vi "Write B.vi"(8 "error in (no error)":errorcluster, 10 "B":dbl, 11 "NumericOperation in":refnum<class "NumericOperation.lvclass">) -> (0 "error out":errorcluster, 3 "NumericOperation out":refnum<class "NumericOperation.lvclass">)   [LabVIEW 2021, in "Calculator.lvlib" / "NumericOperation.lvclass"]
uses:
  NumericOperation.lvclass
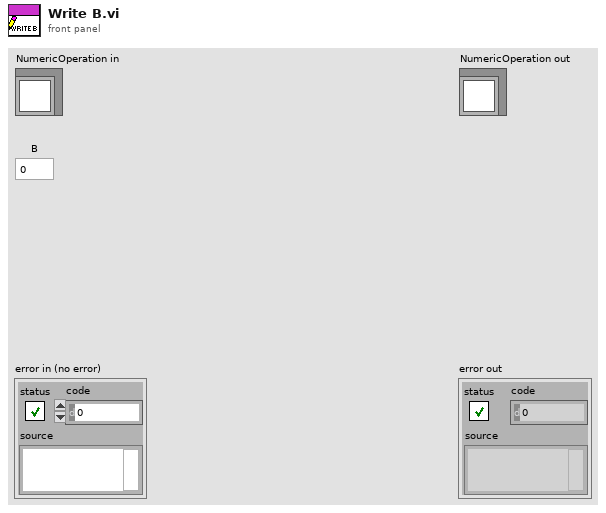
[diagram p1: front panel]
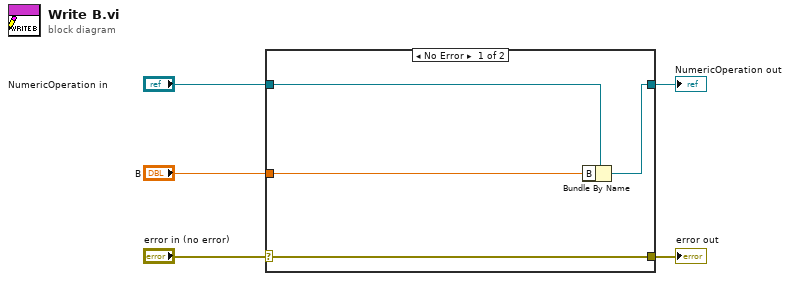
[diagram p0: block diagram]
diagram:
  n1 = case shown="No Error" "error in (no error)" {
    selector: "error in (no error)" -> [w9 w10]
    tunnel: [w9 w10] -> w4
    tunnel: [w7 w11] -> w2
    tunnel: "NumericOperation in" -> [w8 w11]
    tunnel: "B" -> [w6 _]
    frame No Error {
      n2 = Bundle By Name(cluster=w8, "B"=w6) -> (w7:refnum<class "NumericOperation.lvclass">)
    }
    frame Error {
    }
  }
  "error out" <- w4
  "NumericOperation out" <- w2
